vi "8.3.vi"() -> ()   [LabVIEW 2017]
panel:
  out "String":string
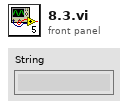
[diagram p1: front panel]
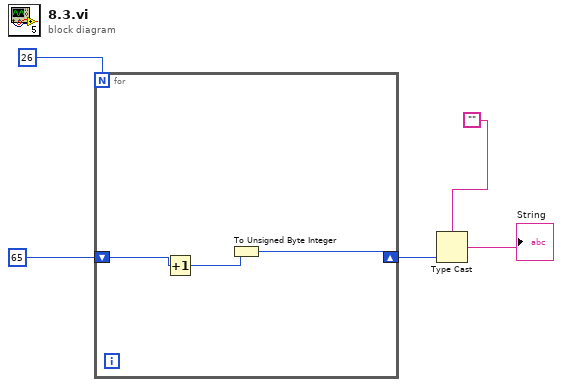
[diagram p0: block diagram]
diagram:
  n1 = for {
    N: 26 -> [_]
    shift-right: [w8] -> w2
    shift-left: 65 -> [w6]
    n2 = Increment(x=w6) -> (x+1=w7:i32)
    n3 = To Unsigned Byte Integer(number=w7) -> (unsigned 8bit integer=w8:u8)
  }
  n4 = Type Cast(type="", x=w2) -> (*(type *) &x=→"String":string)
